vi "Close Messages Refs.vi"(1 "Message Maker in":refnum<class "Message Maker.lvclass">) -> (0 "Message Maker out":refnum<class "Message Maker.lvclass">)   [LabVIEW 2023, in "Message Maker.lvclass"]
uses:
  Message Maker.lvclass
  Message Maker.lvclass/Message Maker.ctl
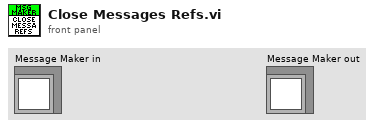
[diagram p1: front panel]
types:
  T1 = typedef "Message Maker.lvclass/Messages Map.ctl" = map{string, T2}
  T2 = typedef "Message Maker.lvclass/Message Details.ctl" = cluster{"Message Ref":refnum<vi>, "Message Type":T3}
  T3 = typedef "Message Maker.lvclass/Message Type.ctl" = enum16{"Standard", "Async"}
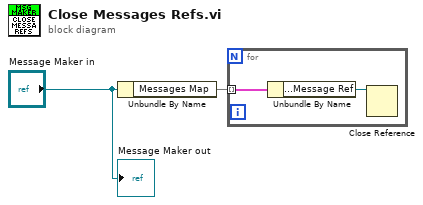
[diagram p0: block diagram]
diagram:
  n1 = Unbundle By Name("Message Maker in") -> ("Messages Map"=w2:T1)
  n2 = for {
    tunnel: w2 -> [w4] mode=indexing
    n3 = Unbundle By Name(w4) -> ("value type.Message Ref"=w3:refnum<vi>)
    n4 = Close Reference(reference=w3) -> ()  [unwired: 1 in, 1 out]
  }
  "Message Maker out" <- "Message Maker in"
